vi "Build Not Equal 0 Compare Types.vi"   [LabVIEW 2021]
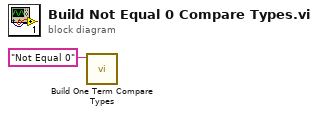
[diagram p0: block diagram]
diagram:
  n1 = call "Build One Term Compare Types.vi"("Comparison Name"="Not Equal 0") -> ()  [unwired: 11 in]
